vi "Gestion_Alarmes.vi"(6 "Numeric":i32, 9 "Numeric 2":i32, 10 "String 2":string, 11 "String":string) -> (1 "y":i32, 2 "Boolean 3":bool, 3 "Boolean 2":bool, 4 "Boolean 4":bool, 5 "Boolean":bool)   [LabVIEW 2026]
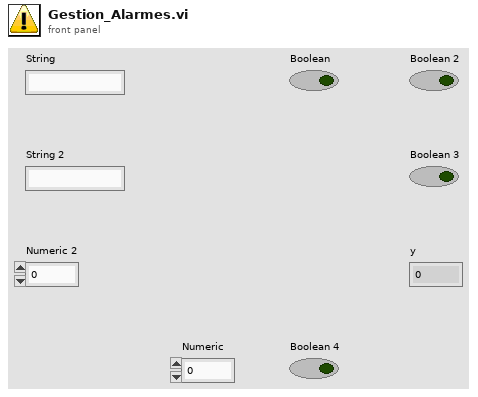
[diagram p1: front panel]
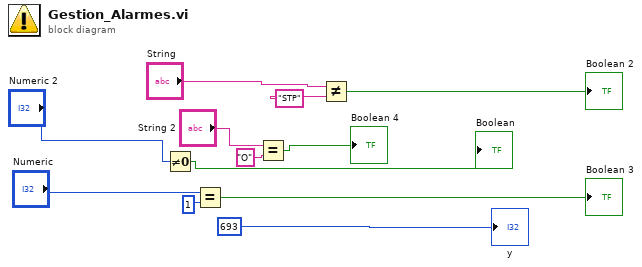
[diagram p0: block diagram]
diagram:
  n1 = Not Equal To 0?(x="Numeric 2") -> (x != 0?=→"Boolean":bool)
  n2 = Equal?(x="Numeric", y=1) -> (x = y?=→"Boolean 3":bool)
  n3 = Equal?(x="String 2", y="O" ("Trames Recues")) -> (x = y?=→"Boolean 4":bool)
  n4 = Not Equal?(x="String", y="STP") -> (x != y?=→"Boolean 2":bool)
  "y" <- 693 ("y")
